vi "DT3120_GetInputSourceList.vi"(8 "error in (no error)":errorcluster, 11 "DevId":i32) -> (0 "error out":errorcluster, 1 "Active Source":u16, 2 "Source List":u16[](array[numeric]), 3 "DevId (dup)":i32)   [LabVIEW 8.6]
uses:
  MT Scan/SubVIs/olfg32.dll
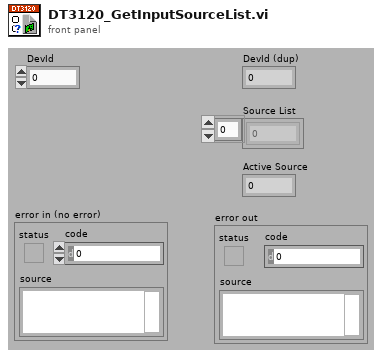
[diagram p1: front panel]
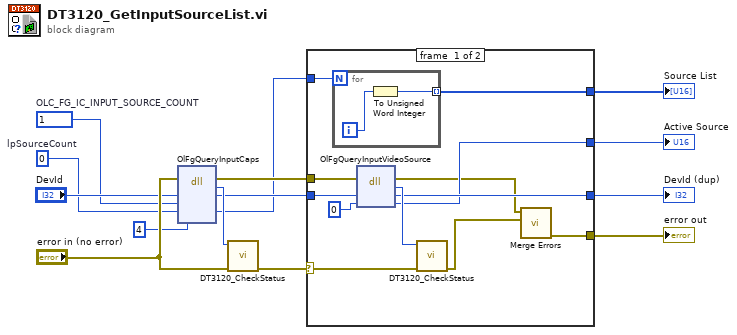
[diagram p0: block diagram]
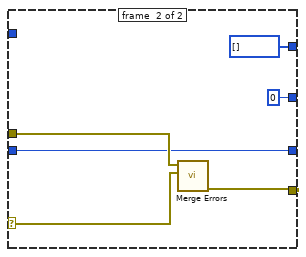
[diagram p2: hidden frame]
diagram:
  w8 = u32 0  # lpSourceCount
  w9 = 1  # OLC_FG_IC_INPUT_SOURCE_COUNT
  n1 = dll-call lib="C:/LabVIEW Programs/MT Scan/SubVIs/olfg32.dll" fn="OlFgQueryInputCaps"(error in="error in (no error)", "DevId"="DevId", "Key"=w9, "lpData"=w8, "DataSize"=u32 4) -> (error out=w12:errorcluster, "Status"=w11:u32, "DevId"=w5:i32, "lpData"=w2:u32)  [unwired: 4 in, 1 out]
  n2 = call "DT3120_CheckStatus.vi"("error in"="error in (no error)", "Status"=w11) -> ("error out"=w6:errorcluster)  [unwired: 9 out]
  n3 = case shown="No Error" w6 {
    selector: w6 -> [w24 w32]
    tunnel: w12 -> [w23 w33]
    tunnel: [w25 w34] -> w14
    tunnel: w5 -> [w21 w31]
    tunnel: [w20 w31] -> w4
    tunnel: [w18 u16 0 ("lpSource")] -> w3
    tunnel: w2 -> [w16 _]
    tunnel: [w15 u16[] []] -> w1
    frame #0 {
      n4 = for {
        N: w16 -> [_]
        tunnel: [w27] -> w15 mode=indexing
        i -> [w28]
        n5 = To Unsigned Word Integer(number=w28) -> (unsigned 16bit integer=w27:u16)
      }
      n6 = dll-call lib="C:/LabVIEW Programs/MT Scan/SubVIs/olfg32.dll" fn="OlFgQueryInputVideoSource"(error in=w23, "DevId"=w21, "lpSource"=u16 0) -> (error out=w17:errorcluster, "Status"=w22:u32, "DevId"=w20:i32, "lpSource"=w18:u16)  [unwired: 2 in, 1 out]
      n7 = call "DT3120_CheckStatus.vi"("error in"=w24, "Status"=w22) -> ("error out"=w26:errorcluster)  [unwired: 2 in, 7 out]
      n8 = call <vilib>:"Merge Errors.vi"("error in 2 (no error)"=w26, "error in 1 (no error)"=w17) -> ("error out"=w25:errorcluster)  [unwired: 2 in, 3 out]
    }
    frame #1 {
      n9 = call <vilib>:"Merge Errors.vi"("error in 2 (no error)"=w32, "error in 1 (no error)"=w33) -> ("error out"=w34:errorcluster)  [unwired: 2 in, 3 out]
    }
  }
  "error out" <- w14
  "DevId (dup)" <- w4
  "Active Source" <- w3
  "Source List" <- w1
